vi "Timeout.vi"(8 "error in (no error)":errorcluster, 10 "Data":variant, 11 "eActor in":refnum<class "eActor.lvclass">) -> (0 "error out":errorcluster, 3 "eActor out":refnum<class "eActor.lvclass">)   [LabVIEW 2015, in "AMS UI.lvlib" / "eActor.lvclass"]
uses:
  eActor.lvclass
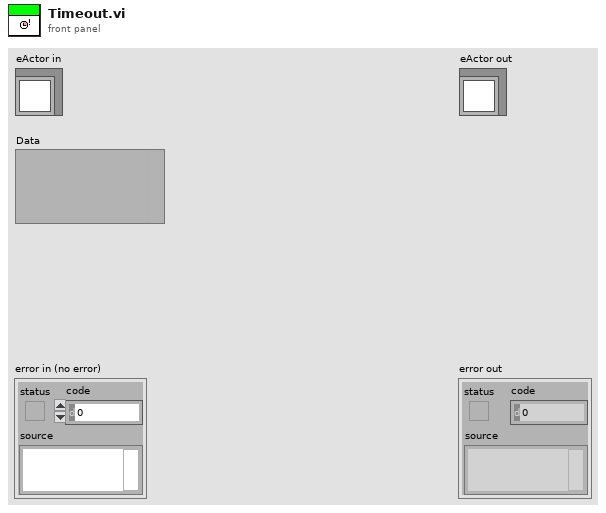
[diagram p1: front panel]
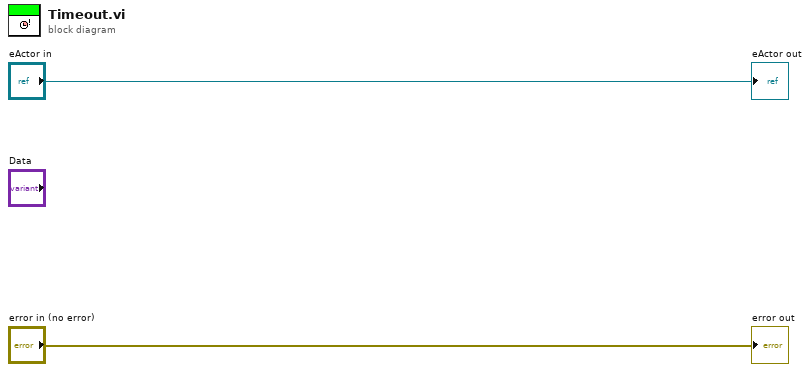
[diagram p0: block diagram]
diagram:
  "error out" <- "error in (no error)"
  "eActor out" <- "eActor in"
